vi "test.vi"() -> ()   [LabVIEW 2014]
panel:
  in  "flashspeed":dbl format="%#_13g"
  in  "intensity":u8=255
  in  "port":i16=32
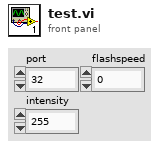
[diagram p1: front panel]
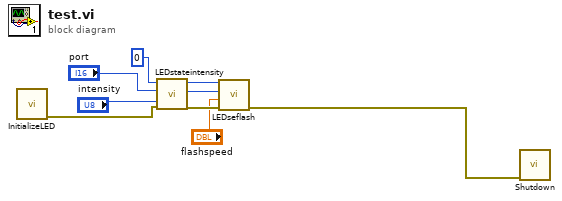
[diagram p0: block diagram]
diagram:
  n1 = call "InitializeLED.vi"() -> ("error out"=w9:errorcluster)  [unwired: 11 in]
  n2 = call "LEDstateintensity.vi"("error in (no error)"=w9, "intensity"="intensity", "port"="port", "Id"=i16 0) -> ("error out"=w5:errorcluster, "port out"=w1:i16, "Id out"=w2:i16)  [unwired: 5 in]
  n3 = call "LEDseflash.vi"("error in (no error)"=w5, "flashspeed"="flashspeed", "port"=w1, "Id"=w2) -> ("error out"=w4:errorcluster)  [unwired: 7 in]
  n4 = call "Shutdown.vi"("error in (no error)"=w4) -> ()  [unwired: 10 in, 1 out]
